vi "DefaultFromIni.vi"(8 "error in (no error)":errorcluster, 11 "MyPluginsBase in":refnum<class "DigitizerBase.lvclass">) -> (0 "error out":errorcluster, 3 "MyPluginsBase out":refnum<class "DigitizerBase.lvclass">)   [LabVIEW 2014, in "DigitizerPlugins.lvlib" / "DigitizerBase.lvclass"]
uses:
  DigitizerBase.lvclass
  Typedefs/Acquisition.ctl
  Typedefs/Trigger.ctl
  Typedefs/TrigSource.ctl
  Typedefs/Channel.ctl
  <userlib>/NIST/BaseClasses/BasePlugin_class/BasePlugin.lvclass/BasePlugin.ctl
  DigitizerBase.lvclass/DigitizerBase.ctl
  <userlib>/NIST/BaseClasses/BasePlugin_class/Accessors/Read PluginIniFilePath.vi
  Accessors/Write Handle.vi
  Accessors/Write Acquisition.vi
  Accessors/Write Trigger.vi
  Accessors/Write Channels.vi
  <vilib>/Utility/config.llb/NI_LVConfig.lvlib
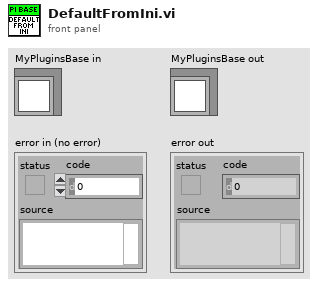
[diagram p1: front panel]
types:
  T1 = typedef "DigitizerPlugins.lvlib/DigitizerBase.lvclass/Channel.ctl" = cluster{"Name":string, "Enabled":bool, "InputImpedance":dbl, "Coupling":enum16{"AC", "DC", "Gnd"}, "Offset":dbl, "Range":dbl}
  T2 = typedef "DigitizerPlugins.lvlib/DigitizerBase.lvclass/Trigger.ctl" = cluster{"Source":string, "Delay":dbl, "Holdoff":dbl, "PretriggerSamples":i32, "Sources":T3[]}
  T3 = typedef "DigitizerPlugins.lvlib/DigitizerBase.lvclass/TrigSource.ctl" = cluster{"Name":string, "Coupling":enum16{"AC", "DC", "HF Reject", "LF Reject", "Noise Reject"}, "Hysteresis":dbl, "Level":dbl, "Slope":enum16{"Positive", "Negative"}, "Type":enum16{"Edge", "Width", "Runt", "Glitch", "TV", "Window"}}
  T4 = typedef "DigitizerPlugins.lvlib/DigitizerBase.lvclass/Acquisition.ctl" = cluster{"SampleRate":dbl, "RecordSize":i32, "NumRecords":i32, "SampleMode":i32, "Timeout (ms)":i32}
  T5 = typedef "NI_LVConfig.lvlib/Config Data RefNum.ctl" = refnum<k1>
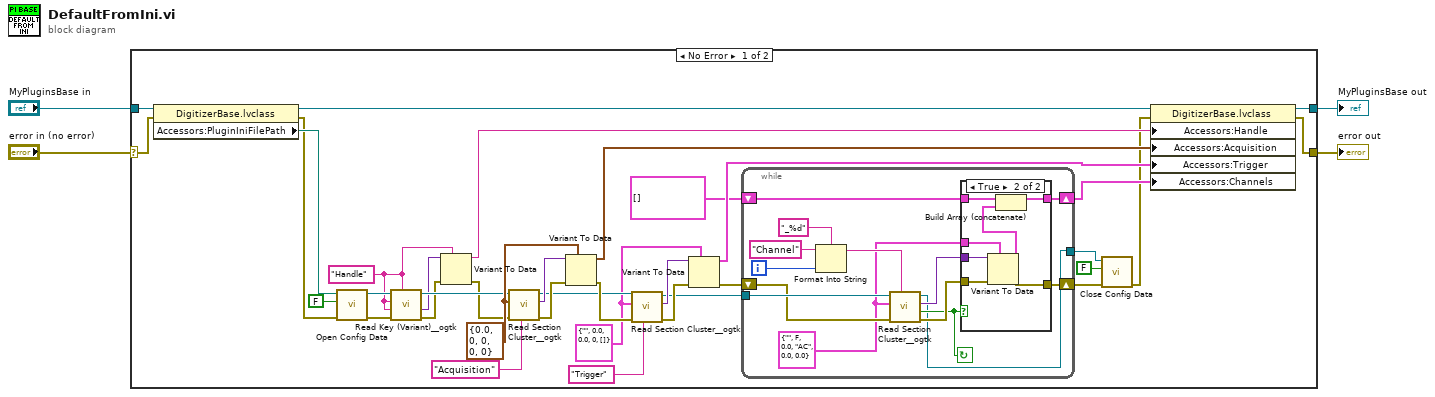
[diagram p0: block diagram]
diagram:
  n1 = case shown="No Error" "error in (no error)" {
    selector: "error in (no error)" -> [w38 w65]
    tunnel: [w20 w65] -> w3
    tunnel: [w37 w64] -> w1
    tunnel: "MyPluginsBase in" -> [w40 w64]
    frame No Error {
      w13 = "Handle" ("section")
      w24 = T2 {"Source"="", "Delay"=0.0, "Holdoff"=0.0, "PretriggerSamples"=0, "Sources"=[]} ("Trigger")
      w31 = T4 {"SampleRate"=0.0, "RecordSize"=0, "NumRecords"=0, "SampleMode"=0, "Timeout (ms)"=0} ("Acquisition")
      n2 = property class="DigitizerBase.lvclass"(reference=w40, error in=w38) -> (reference out=w39:refnum<class "DigitizerBase.lvclass">, error out=w35:errorcluster, "Accessors:PluginIniFilePath"=w36:path)
      n3 = call <vilib>:"Open Config Data.vi"("error in (no error)"=w35, "create file if necessary (T)"=FALSE, "configuration file path"=w36) -> ("error out"=w17:errorcluster, "refnum"=w16:T5)  [unwired: 6 in, 1 out]
      n4 = call <userlib>:"Read Key (Variant)__ogtk.vi"("section"=w13, "error in (no error)"=w17, "type"=w13, "key (optional)"=w13, "refnum"=w16) -> ("error out"=w11:errorcluster, "key-value"=w12:variant, "refnum out"=w14:T5)  [unwired: 3 in, 1 out]
      n5 = Variant To Data(error in=w11, type=w13, Variant=w12) -> (data=w9:string, error out=w10:errorcluster)
      n6 = call <userlib>:"Read Section Cluster__ogtk.vi"("section (optional)"="Acquisition", "error in (no error)"=w10, "Section Formatted Cluster Type"=w31, "refnum"=w14) -> ("error out"=w30:errorcluster, "Section Formatted Cluster"=w32:variant, "dup refnum"=w27:T5)  [unwired: 3 in, 2 out]
      n7 = Variant To Data(error in=w30, type=w31, Variant=w32) -> (data=w15:T4, error out=w28:errorcluster)
      n8 = call <userlib>:"Read Section Cluster__ogtk.vi"("section (optional)"="Trigger", "error in (no error)"=w28, "Section Formatted Cluster Type"=w24, "refnum"=w27) -> ("error out"=w25:errorcluster, "Section Formatted Cluster"=w29:variant, "dup refnum"=w23:T5)  [unwired: 3 in, 2 out]
      n9 = Variant To Data(error in=w25, type=w24, Variant=w29) -> (data=w21:T2, error out=w22:errorcluster)
      n10 = while {
        tunnel: w23 -> [w50]
        shift-right: [w45] -> w8
        shift-left: w22 -> [w49]
        shift-right: [w43] -> w18
        shift-left: T1[] [] ("Channels") -> [w44]
        tunnel: [w41] -> w7
        i -> [w52]
        stop <- w42 continue-if-true
        w46 = T1 {"Name"="", "Enabled"=FALSE, "InputImpedance"=0.0, "Coupling"=enum."AC", "Offset"=0.0, "Range"=0.0} ("Channel")
        n11 = Format Into String(format string="_%d", initial string="Channel" ("section (optional)"), w52) -> (resulting string=w51:string)  [unwired: 1 in, 1 out]
        n12 = call <userlib>:"Read Section Cluster__ogtk.vi"("section (optional)"=w51, "error in (no error)"=w49, "Section Formatted Cluster Type"=w46, "refnum"=w50) -> ("error out"=w47:errorcluster, "all found?"=w42:bool, "Section Formatted Cluster"=w48:variant, "dup refnum"=w41:T5)  [unwired: 3 in, 1 out]
        n13 = case shown="True" w42 {
          tunnel: w48 -> [_ w63]
          tunnel: w47 -> [w55 w62]
          tunnel: w46 -> [_ w61]
          tunnel: [w55 w60] -> w45
          tunnel: w44 -> [w56 w59]
          tunnel: [w56 w58] -> w43
          frame False {
          }
          frame True {
            n14 = Variant To Data(error in=w62, type=w61, Variant=w63) -> (data=w57:T1, error out=w60:errorcluster)
            n15 = Build Array (concatenate)(w59, w57) -> (w58:T1[])
          }
        }
      }
      n16 = call <vilib>:"Close Config Data.vi"("error in (no error)"=w8, "write file if changed (T)"=FALSE, "refnum"=w7) -> ("error out"=w5:errorcluster)  [unwired: 7 in, 1 out]
      n17 = property class="DigitizerBase.lvclass"(reference=w39, error in=w5, "Accessors:Handle"=w9, "Accessors:Acquisition"=w15, "Accessors:Trigger"=w21, "Accessors:Channels"=w18) -> (reference out=w37:refnum<class "DigitizerBase.lvclass">, error out=w20:errorcluster)
    }
    frame Error {
    }
  }
  "error out" <- w3
  "MyPluginsBase out" <- w1
